vi "_TestONRegion.vi"(0 "VISA Resource Name":refnum<visa-resource-name>, 1 "Project #":string, 2 "Request #":string, 3 "TEST #":string, 4 "ICE":dbl, 5 "VGE":dbl, 6 "VCE":dbl, 7 "error in (no error)":errorcluster) -> (8 "Tdon (ns)":dbl, 9 "Di (A)":dbl, 10 "Tr (ns)":dbl, 11 "Dt (ns)":dbl, 12 "Di/Dt (A/us)":dbl, 14 "Dv/Dt (V/us)":dbl, 16 "Eon (uj)":dbl, 17 "Dv (V)":dbl, 19 "Dt (ns) 2":dbl, 20 "DONE Tdon":bool, 21 "DONE Tr":bool, 22 "DONE Di/Dt ON":bool, 23 "DONE Dv/Dt ON":bool, 24 "DONE Eon":bool, 26 "Waveform Graph":waveform(dbl)[](graph), 27 "error out":errorcluster)   [LabVIEW 2020]
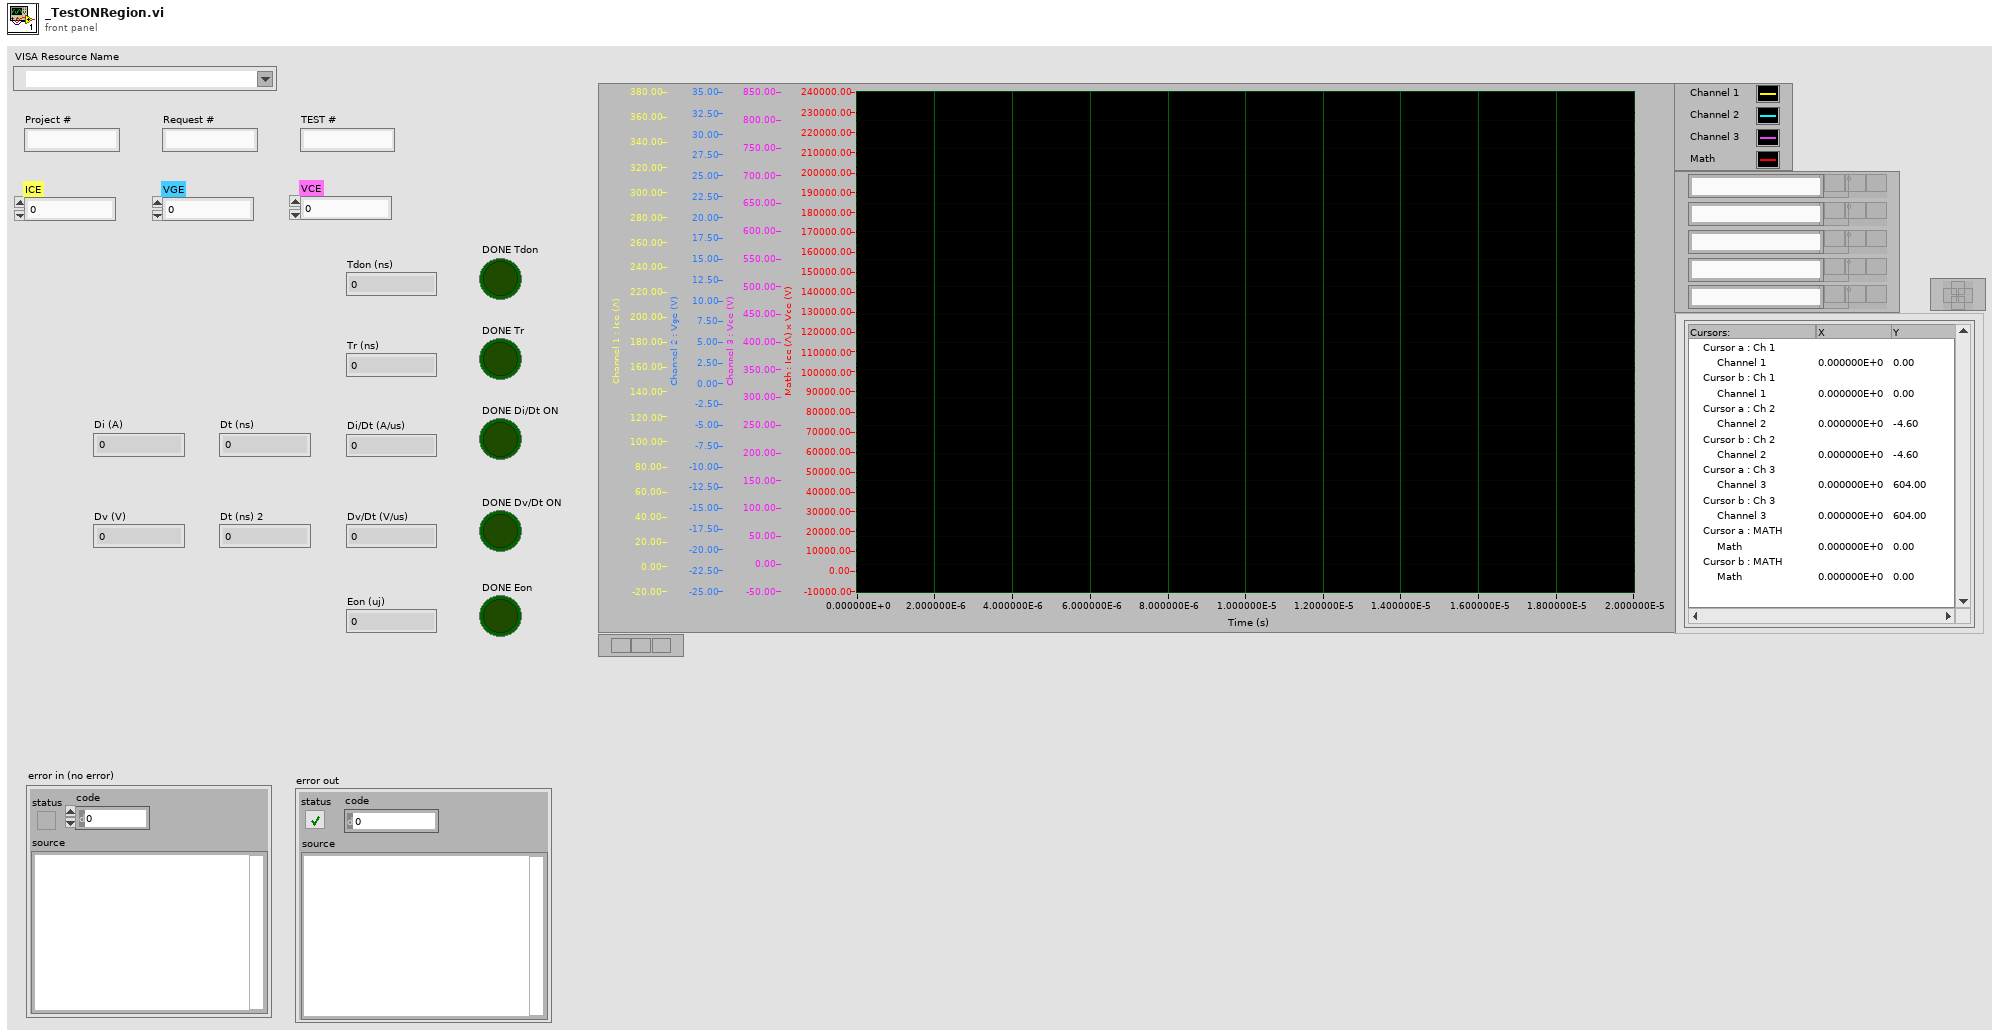
[diagram p1: front panel]
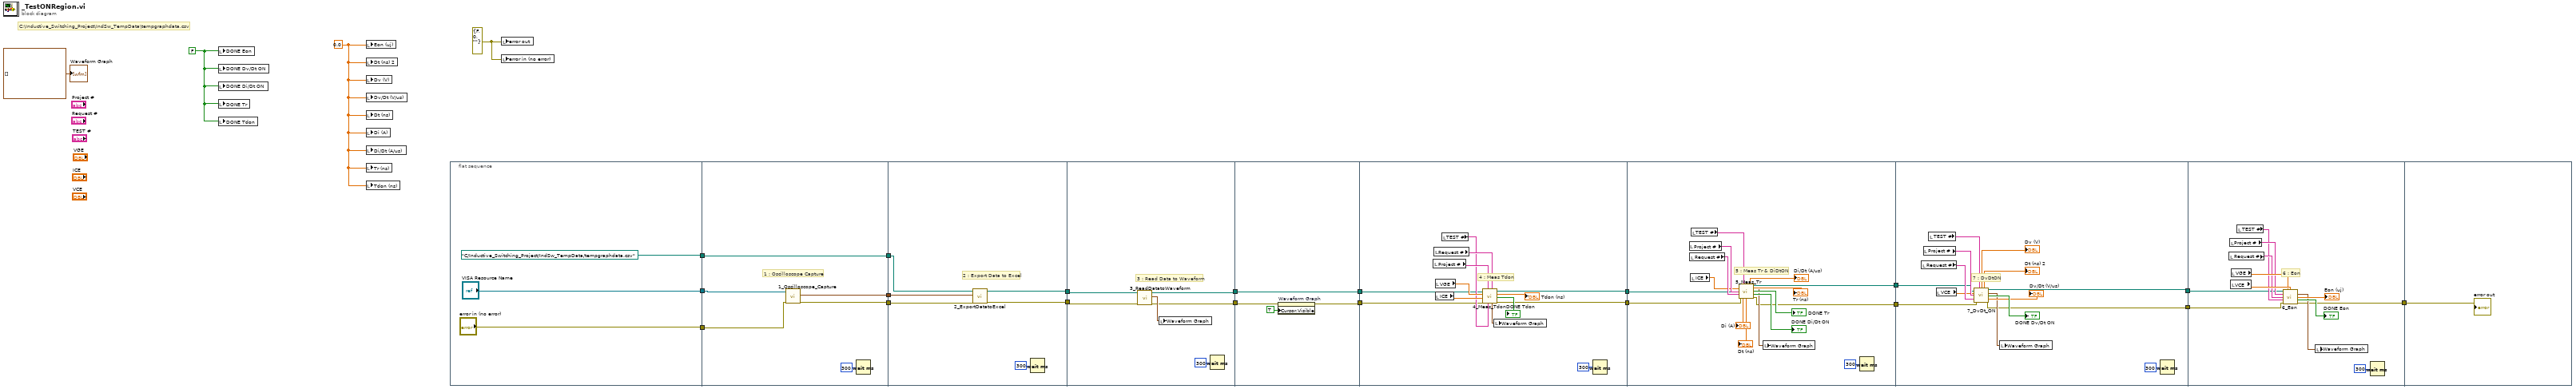
[diagram p0: block diagram]
diagram:
  w4 = errorcluster {"status"=FALSE, "code"=0, "source"=""} ("error out")
  w21 = 0.0 ("Eon (uj)")
  w22 = FALSE ("DONE Eon")
  # "C:\\Inductive_Switching_Project\\IndSw_TempData\\tempgraphdata.csv"
  n1 = local write "DONE Eon"(w22) -> ()
  n2 = local write "DONE Dv/Dt ON"(w22) -> ()
  n3 = local write "DONE Di/Dt ON"(w22) -> ()
  n4 = local write "DONE Tr"(w22) -> ()
  n5 = local write "DONE Tdon"(w22) -> ()
  n6 = local write "Eon (uj)"(w21) -> ()
  n7 = local write "Dt (ns) 2"(w21) -> ()
  n8 = local write "Dv (V)"(w21) -> ()
  n9 = local write "Dv/Dt (V/us)"(w21) -> ()
  n10 = local write "Dt (ns)"(w21) -> ()
  n11 = local write "Di (A)"(w21) -> ()
  n12 = local write "Di/Dt (A/us)"(w21) -> ()
  n13 = local write "Tr (ns)"(w21) -> ()
  n14 = local write "Tdon (ns)"(w21) -> ()
  n15 = flat-sequence {
    tunnel: [path "C:/Inductive_Switching_Project/IndSw_TempData/tempgraphdata.csv" ("file path (IN)")] -> w3
    tunnel: ["error in (no error)"] -> w2
    tunnel: ["VISA Resource Name"] -> w1
    tunnel: [w29] -> w11
    tunnel: [w28] -> w10
    tunnel: [w32] -> w9
    tunnel: w3 -> [w32]
    tunnel: w2 -> [w31]
    tunnel: w1 -> [w30]
    tunnel: [w35] -> w13
    tunnel: [w34] -> w12
    tunnel: w11 -> [w38]
    tunnel: w10 -> [w37]
    tunnel: w9 -> [w36]
    tunnel: [w41] -> w8
    tunnel: [w40] -> w6
    tunnel: w13 -> [w43]
    tunnel: w12 -> [w42]
    tunnel: w8 -> [w47]
    tunnel: [w46] -> w7
    tunnel: w6 -> [w48]
    tunnel: [w48] -> w5
    tunnel: [w50] -> w15
    tunnel: [w51] -> w14
    tunnel: w7 -> [w53]
    tunnel: w5 -> [w52]
    tunnel: [w64] -> w17
    tunnel: [w63] -> w16
    tunnel: w15 -> [w66]
    tunnel: w14 -> [w65]
    tunnel: [w80] -> w19
    tunnel: [w79] -> w18
    tunnel: w17 -> [w82]
    tunnel: w16 -> [w81]
    tunnel: [w93] -> w20
    tunnel: w19 -> [w95]
    tunnel: w18 -> [w94]
    tunnel: w20 -> [w104]
    frame #0 {
    }
    frame #1 {
      # "1 : Oscilloscope Capture"
      n16 = call "1_Oscilloscope_Capture.vi"("error in (no error)"=w31, "VISA Resource Name"=w30) -> ("error out"=w29:errorcluster, "Waveform Graph"=w28:waveform(dbl)[])  [unwired: 7 in, 1 out]
      n17 = Wait (ms)(milliseconds to wait=u32 300) -> ()  [unwired: 1 out]
    }
    frame #2 {
      # "2 : Export Data to Excel"
      n18 = call "2_ExportDatatoExcel.vi"("error in (no error)"=w38, "Waveform Graph"=w37, "file path (IN)"=w36) -> ("error out"=w35:errorcluster, "file path (OUT)"=w34:path)  [unwired: 7 in]
      n19 = Wait (ms)(milliseconds to wait=u32 300) -> ()  [unwired: 1 out]
    }
    frame #3 {
      # "3 : Read Data to Waveform"
      n20 = call "3_ReadDatatoWaveform.vi"("error in (no error)"=w43, "file path (IN)"=w42) -> ("error out"=w41:errorcluster, "Waveform Graph"=w44:waveform(dbl)[], "file path (OUT)"=w40:path)  [unwired: 3 in, 4 out]
      n21 = local write "Waveform Graph"(w44) -> ()
      n22 = Wait (ms)(milliseconds to wait=u32 300) -> ()  [unwired: 1 out]
    }
    frame #4 {
      n23 = property on="Waveform Graph" class="WFGraph (strict)"(error in=w47, "Cursor.Visible"=TRUE) -> (error out=w46:errorcluster)  [unwired: 1 in, 1 out]
    }
    frame #5 {
      # "4 : Meas Tdon"
      n24 = local read "Project #"() -> (w58:string)
      n25 = local read "Request #"() -> (w59:string)
      n26 = local read "VGE"() -> (w60:dbl)
      n27 = local read "ICE"() -> (w61:dbl)
      n28 = local read "TEST #"() -> (w57:string)
      n29 = call "4_Meas_Tdon.vi"("Request #"=w59, "TEST #"=w57, "Project #"=w58, "error in (no error)"=w53, "ICE"=w61, "VGE"=w60, "file path (IN)"=w52) -> ("error out"=w51:errorcluster, "DONE Tdon"=→"DONE Tdon":bool, "Tdon (ns)"=→"Tdon (ns)":dbl, "file path (OUT)"=w50:path, "ON Region"=w54:waveform(dbl)[])
      n30 = local write "Waveform Graph"(w54) -> ()
      n31 = Wait (ms)(milliseconds to wait=u32 300) -> ()  [unwired: 1 out]
    }
    frame #6 {
      # "5 : Meas Tr & DiDtON"
      n32 = local read "Project #"() -> (w69:string)
      n33 = local read "Request #"() -> (w70:string)
      n34 = local read "ICE"() -> (w68:dbl)
      n35 = local read "TEST #"() -> (w71:string)
      n36 = call "5_Meas_Tr.vi"("file path (IN)"=w66, "TEST #"=w71, "ICE"=w68, "Project #"=w69, "Request #"=w70, "error in (no error)"=w65) -> ("Tr (ns)"=→"Tr (ns)":dbl, "Di/Dt (A/us)"=→"Di/Dt (A/us)":dbl, "file path (OUT)"=w64:path, "ON Region"=w67:waveform(dbl)[], "DONE Tr"=→"DONE Tr":bool, "DONE Di/Dt ON"=→"DONE Di/Dt ON":bool, "Di (A)"=→"Di (A)":dbl, "Dt (ns)"=→"Dt (ns)":dbl, "error out"=w63:errorcluster)  [unwired: 1 in]
      n37 = local write "Waveform Graph"(w67) -> ()
      n38 = Wait (ms)(milliseconds to wait=u32 300) -> ()  [unwired: 1 out]
    }
    frame #7 {
      # "7 : DvDtON"
      n39 = local read "Request #"() -> (w87:string)
      n40 = local read "Project #"() -> (w86:string)
      n41 = local read "TEST #"() -> (w85:string)
      n42 = local read "VCE"() -> (w84:dbl)
      n43 = call "7_DvDt_ON.vi"("file path (IN)"=w82, "TEST #"=w85, "VCE"=w84, "Project #"=w86, "Request #"=w87, "error in (no error)"=w81) -> ("Dv (V)"=→"Dv (V)":dbl, "Dt (ns)"=→"Dt (ns) 2":dbl, "file path (OUT)"=w80:path, "ON Region"=w83:waveform(dbl)[], "DONE Dv/Dt ON"=→"DONE Dv/Dt ON":bool, "Dv/Dt (V/us)"=→"Dv/Dt (V/us)":dbl, "error out"=w79:errorcluster)  [unwired: 3 in]
      n44 = local write "Waveform Graph"(w83) -> ()
      n45 = Wait (ms)(milliseconds to wait=u32 300) -> ()  [unwired: 1 out]
    }
    frame #8 {
      # "6 : Eon"
      n46 = local read "Request #"() -> (w99:string)
      n47 = local read "Project #"() -> (w98:string)
      n48 = local read "VCE"() -> (w101:dbl)
      n49 = local read "VGE"() -> (w100:dbl)
      n50 = local read "TEST #"() -> (w97:string)
      n51 = call "6_Eon.vi"("file path (IN)"=w95, "VGE"=w100, "VCE"=w101, "Project #"=w98, "Request #"=w99, "TEST #"=w97, "error in (no error)"=w94) -> ("ON Region"=w96:waveform(dbl)[], "Eon (uj)"=→"Eon (uj)":dbl, "DONE Eon"=→"DONE Eon":bool, "error out"=w93:errorcluster)  [unwired: 4 in, 1 out]
      n52 = local write "Waveform Graph"(w96) -> ()
      n53 = Wait (ms)(milliseconds to wait=u32 300) -> ()  [unwired: 1 out]
    }
    frame #9 {
      "error out" <- w104
    }
  }
  n54 = local write "error out"(w4) -> ()
  n55 = local write "error in (no error)"(w4) -> ()
  "Waveform Graph" <- waveform(dbl)[] [] ("Waveform Graph")
